vi "Collector.vi"(6 "MotorSpeed":dbl, 7 "Action":T10, 8 "Error in":errorcluster, 9 "BottomLS":T8={"DevStatus"={"status"=FALSE, "code"=0, "source"=""}, "DIO Channel"=enum."Invalid", "Digital Module"=enum."Digital Module 1"}, 10 "TopLS":T8={"DevStatus"={"status"=FALSE, "code"=0, "source"=""}, "DIO Channel"=enum."Invalid", "Digital Module"=enum."Digital Module 1"}, 11 "Motor":T1={"DeviceStatus"={"status"=FALSE, "code"=0, "source"=""}, "Type"=enum."PWM", "PWM"={"Digital Module"=enum."Digital Module 1", "PWM Channel"=enum."Invalid", "DeadBand"={"Name"="", "maxPositivePwm"=0, "minPositivePwm"=0, "centerPwm"=0, "maxNegativePwm"=0, "minNegativePwm"=0, "angularRange"=0}}, "CAN"={"Device Number"=0, "Control Mode"=enum."Percent VBus", "Semaphore"=refnum, "Max Vout"=12.0}, "Invert"=FALSE, "TransformRef"=refnum, "InvTransformRef"=refnum}) -> (0 "Error out":errorcluster, 1 "Lower Triggered?":bool, 2 "Upper Triggered?":bool)   [LabVIEW 2013]
doc: "Controls the collector arm, along with the two sets of limit switches associated with it (one set all the way up, the other all the way down). NOTE: all states return the status of the limit switches. It has the following actions:\n-Init: takes references to the motor and limit switches and stores them in shift registers\n-Raise: attempts to raise the collector (nothing happens if the upper limit switch is triggered)\n-Lower: attempts to lower the collector (nothing happens if the lower limit switch is triggered)\n-Stop: stops the motor\n-GetStatus: returns the value of the limit switches"
uses:
  CollectorAction.ctl
  <vilib>/Rock Robotics/WPI/DigitalInput/WPI_DigitalInputDevRef.ctl
  <vilib>/Rock Robotics/SystemInterfaces/DIO/FPGA_DIOChannel.ctl
  <vilib>/Rock Robotics/SystemInterfaces/Typedef/FPGA_TypedefDigitalModule.ctl
  <vilib>/Rock Robotics/WPI/MotorControl/WPI_MotorControlDeviceRef.ctl
  <vilib>/Rock Robotics/SystemInterfaces/DIO/FPGA_DIOPWMChannel.ctl
  <vilib>/Rock Robotics/WPI/PWM/WPI_PWMDeadband.ctl
  <vilib>/Rock Robotics/WPI/CAN/Jaguar/SubVIs/WPI_CANJaguar_ControlMode.ctl
  <vilib>/Rock Robotics/WPI/PWM/WPI_PWMTransform_ConPane.ctl
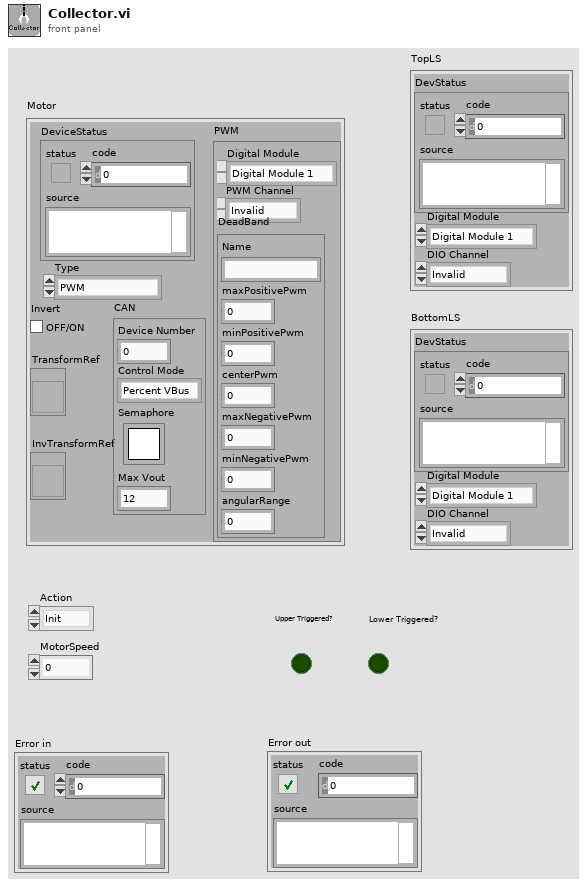
[diagram p1: front panel]
types:
  T1 = typedef "WPI_MotorControlDeviceRef.ctl" = cluster{"DeviceStatus":errorcluster, "Type":enum16{"PWM", "CAN"}, "PWM":cluster{"Digital Module":T2, "PWM Channel":T3, "DeadBand":T4}, "CAN":cluster{"Device Number":u8, "Control Mode":T5, "Semaphore":T6, "Max Vout":dbl}, "Invert":bool, "TransformRef":T7, "InvTransformRef":T7}
  T2 = typedef "FPGA_TypedefDigitalModule.ctl" = enum16{"Digital Module 1", "Digital Module 2"}
  T3 = typedef "FPGA_DIOPWMChannel.ctl" = enum8{"PWM 1", "PWM 2", "PWM 3", "PWM 4", "PWM 5", "PWM 6", "PWM 7", "PWM 8", "PWM 9", "PWM 10", "Invalid"}
  T4 = typedef "WPI_PWMDeadband.ctl" = cluster{"Name":string, "maxPositivePwm":i32, "minPositivePwm":i32, "centerPwm":i32, "maxNegativePwm":i32, "minNegativePwm":i32, "angularRange":u16}
  T5 = typedef "WPI_CANJaguar_ControlMode.ctl" = enum8{"Percent VBus", "Current", "Speed", "Position", "Voltage"}
  T6 = typedef "Semaphore RefNum" = refnum<k1>
  T7 = typedef "WPI_PWMTransform_ConPane.ctl" = refnum<vi>
  T8 = typedef "WPI_DigitalInputDevRef.ctl" = cluster{"DevStatus":errorcluster, "DIO Channel":T9, "Digital Module":T2}
  T9 = typedef "FPGA_DIOChannel.ctl" = enum8{"DIO 1", "DIO 2", "DIO 3", "DIO 4", "DIO 5", "DIO 6", "DIO 7", "DIO 8", "DIO 9", "DIO 10", "DIO 11", "DIO 12", "DIO 13", "DIO 14", "Invalid"}
  T10 = typedef "CollectorAction.ctl" = enum16{"Init", "Raise", "Lower", "Stop", "GetStatus"}
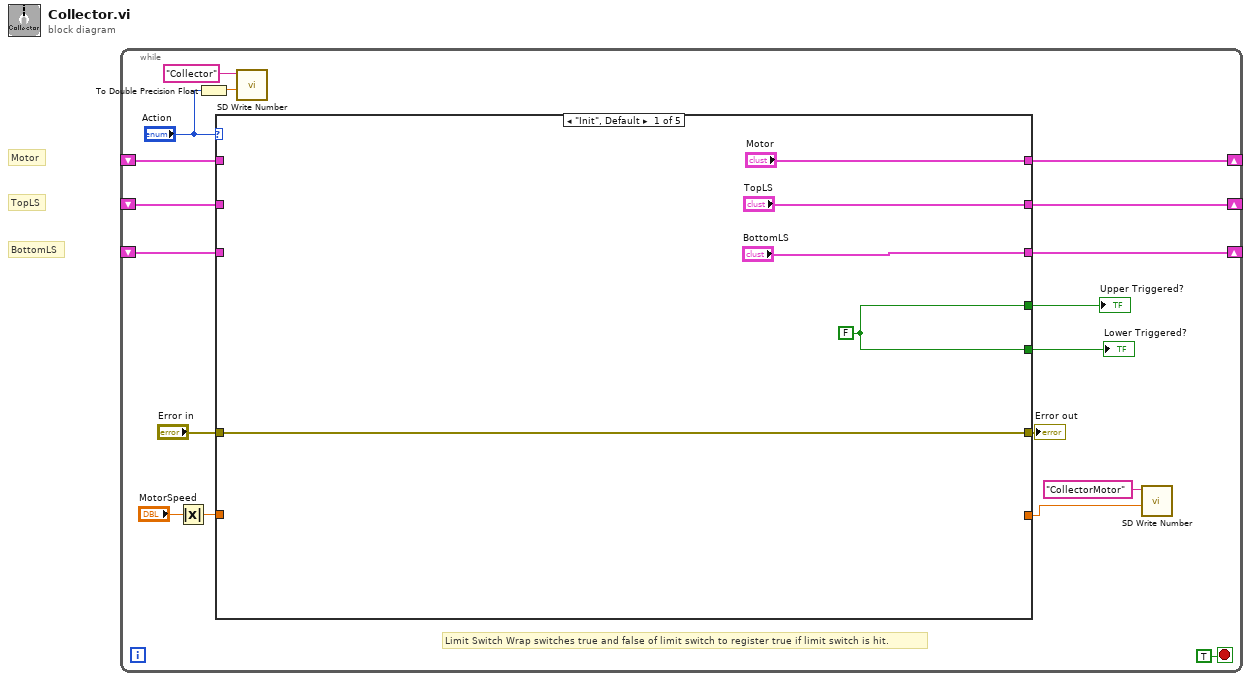
[diagram p0: block diagram]
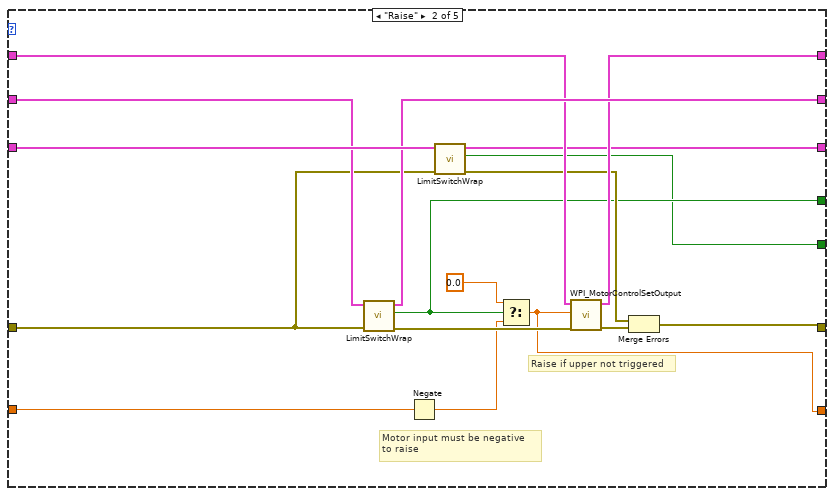
[diagram p2: hidden frame]
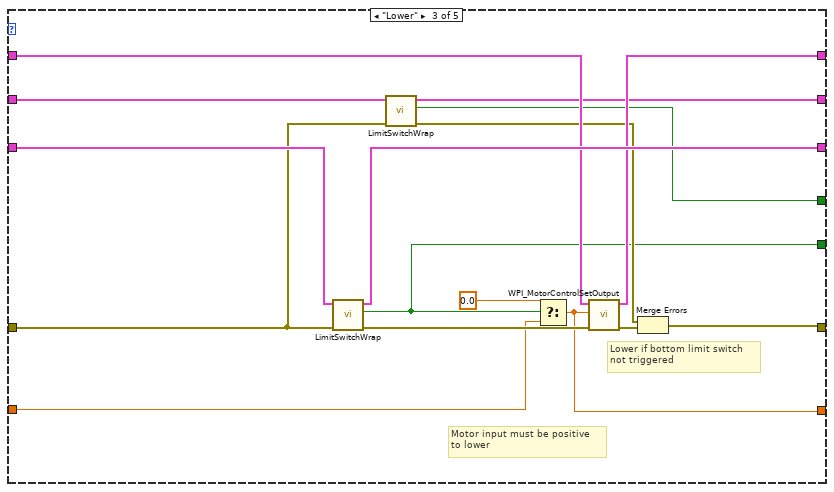
[diagram p3: hidden frame]
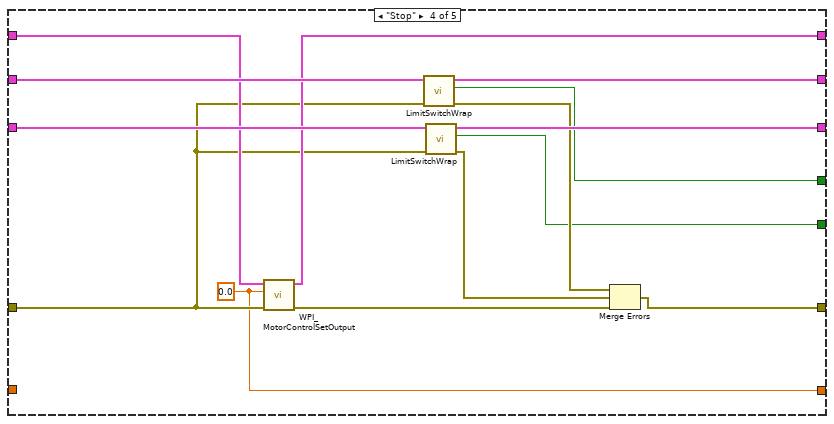
[diagram p4: hidden frame]
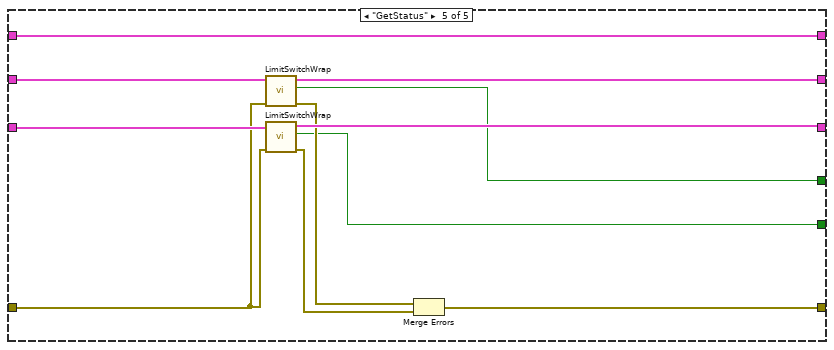
[diagram p5: hidden frame]
diagram:
  # "BottomLS"
  # "TopLS"
  # "Motor"
  n1 = while {
    shift-right: [w15] -> _
    shift-left: _ -> [w12]
    shift-right: [w16] -> _
    shift-left: _ -> [w13]
    shift-right: [w17] -> _
    shift-left: _ -> [w14]
    stop <- TRUE stop-if-true
    # "Limit Switch Wrap switches true and false of limit switch to register true if limit switch is hit."
    n2 = Absolute Value(x="MotorSpeed") -> (abs(x)=w6:dbl)
    n3 = To Double Precision Float(number="Action") -> (double precision float=w3:dbl)
    n4 = case shown="\"Init\", Default" "Action" {
      tunnel: ["Motor" w34 w50 w67 w81] -> w17
      tunnel: ["TopLS" w36 w49 w65 w78] -> w16
      tunnel: ["BottomLS" w33 w53 w66 w77] -> w15
      tunnel: w14 -> [_ w35 w51 w68 w81]
      tunnel: w13 -> [_ w37 w56 w70 w79]
      tunnel: w12 -> [_ w40 w54 w69 w80]
      tunnel: "Error in" -> [w23 w32 w48 w64 w76]
      tunnel: [w23 w30 w47 w62 w73] -> w10
      tunnel: [w19 w27 w43 w59 w72] -> w8
      tunnel: [w19 w28 w44 w58 w71] -> w9
      tunnel: w6 -> [_ w26 w42 _ _]
      tunnel: [_ w24 w41 w57 _] -> w1
      frame "Init", Default {
        w19 = FALSE
      }
      frame "Raise" {
        # "Motor input must be negative\nto raise"
        # "Raise if upper not triggered"
        n5 = call "LimitSwitchWrap.vi"("error in"=w32, "DigitalInputDevRef"=w37) -> ("error out"=w38:errorcluster, "Triggered"=w28:bool, "DigitalInputDevRef 2"=w36:T8)  [unwired: 7 in]
        n6 = Negate(x=w26) -> (-x=w25:dbl)
        n7 = call "LimitSwitchWrap.vi"("error in"=w32, "DigitalInputDevRef"=w40) -> ("error out"=w29:errorcluster, "Triggered"=w27:bool, "DigitalInputDevRef 2"=w33:T8)  [unwired: 7 in]
        n8 = Select(t=0.0, s=w28, f=w25) -> (s? t:f=w24:dbl)
        n9 = call <vilib>:"WPI_MotorControlSetOutput.vi"("error in (no error)"=w38, "Output"=w24, "MotorControlDevRef"=w35) -> ("error out"=w31:errorcluster, "MotorControlDevRef"=w34:T1)  [unwired: 6 in, 1 out]
        n10 = Merge Errors(w29, w31) -> (w30:errorcluster)
      }
      frame "Lower" {
        # "Motor input must be positive\nto lower"
        # "Lower if bottom limit switch\nnot triggered"
        n11 = call "LimitSwitchWrap.vi"("error in"=w48, "DigitalInputDevRef"=w54) -> ("error out"=w52:errorcluster, "Triggered"=w43:bool, "DigitalInputDevRef 2"=w53:T8)  [unwired: 7 in]
        n12 = call "LimitSwitchWrap.vi"("error in"=w48, "DigitalInputDevRef"=w56) -> ("error out"=w45:errorcluster, "Triggered"=w44:bool, "DigitalInputDevRef 2"=w49:T8)  [unwired: 7 in]
        n13 = Select(t=0.0, s=w43, f=w42) -> (s? t:f=w41:dbl)
        n14 = call <vilib>:"WPI_MotorControlSetOutput.vi"("error in (no error)"=w52, "Output"=w41, "MotorControlDevRef"=w51) -> ("error out"=w46:errorcluster, "MotorControlDevRef"=w50:T1)  [unwired: 6 in, 1 out]
        n15 = Merge Errors(w45, w46) -> (w47:errorcluster)
      }
      frame "Stop" {
        w57 = 0.0
        n16 = call <vilib>:"WPI_MotorControlSetOutput.vi"("error in (no error)"=w64, "Output"=w57, "MotorControlDevRef"=w68) -> ("error out"=w63:errorcluster, "MotorControlDevRef"=w67:T1)  [unwired: 6 in, 1 out]
        n17 = call "LimitSwitchWrap.vi"("error in"=w64, "DigitalInputDevRef"=w70) -> ("error out"=w60:errorcluster, "Triggered"=w58:bool, "DigitalInputDevRef 2"=w65:T8)  [unwired: 7 in]
        n18 = call "LimitSwitchWrap.vi"("error in"=w64, "DigitalInputDevRef"=w69) -> ("error out"=w61:errorcluster, "Triggered"=w59:bool, "DigitalInputDevRef 2"=w66:T8)  [unwired: 7 in]
        n19 = Merge Errors(w60, w61, w63) -> (w62:errorcluster)
      }
      frame "GetStatus" {
        n20 = call "LimitSwitchWrap.vi"("error in"=w76, "DigitalInputDevRef"=w79) -> ("error out"=w74:errorcluster, "Triggered"=w71:bool, "DigitalInputDevRef 2"=w78:T8)  [unwired: 7 in]
        n21 = call "LimitSwitchWrap.vi"("error in"=w76, "DigitalInputDevRef"=w80) -> ("error out"=w75:errorcluster, "Triggered"=w72:bool, "DigitalInputDevRef 2"=w77:T8)  [unwired: 7 in]
        n22 = Merge Errors(w74, w75) -> (w73:errorcluster)
      }
    }
    "Error out" <- w10
    "Upper Triggered?" <- w9
    "Lower Triggered?" <- w8
    n23 = call <vilib>:"SD Write Number.vi"("Numeric"=w3, "Name"="Collector") -> ()  [unwired: 8 in, 2 out]
    n24 = call <vilib>:"SD Write Number.vi"("Numeric"=w1, "Name"="CollectorMotor") -> ()  [unwired: 8 in, 2 out]
  }
